vi "systemid-hardware-analyzer.vi"() -> ()   [LabVIEW 2012]
uses:
  <vilib>/addons/Control Design/_Utility/Model Viewer.llb/Model Viewer SubVI/cd_Draw Zero-Pole-Gain Equation (ZPK).vi
  <vilib>/imath/engines/lvmath2/RunTimeEngine/ErrorHandling/NIMS_Finalize Error.vi
  <vilib>/imath/engines/lvmath2/RunTimeEngine/Managers/WorkSpace/UID Generator.vi
  <vilib>/imath/engines/lvmath/Plug In/_Char/NIMS_CH_U8 2D to Character 2D.vi
  <vilib>/imath/engines/lvmath/Plug In/_Char/NIMS_CH_Character 2D to String 1D.vi
  <vilib>/imath/engines/lvmath2/RunTimeEngine/NodeEndStatement/NIMS_NodeEndStatement_Get Scalar.vi
  <instcachedir>/0/NIMS_NodeEndStatement_Get Scalar_DDDE03B66C1B40AEB228387CE0451FA8.lvgen/NIMS_NodeEndStatement_Get Scalar_DDDE03B66C1B40AEB228387CE0451FA8_000.vi
  <vilib>/imath/engines/lvmath2/RunTimeEngine/NodeEndStatement/NIMS_NodeEndStatement_Get Vector.vi
  <instcachedir>/0/NIMS_NodeEndStatement_Get Vector_2BE3967F82A04EDB90B65AFAEF9E88C9.lvgen/NIMS_NodeEndStatement_Get Vector_2BE3967F82A04EDB90B65AFAEF9E88C9_001.vi
  <instcachedir>/0/NIMS_NodeEndStatement_Get Vector_2BE3967F82A04EDB90B65AFAEF9E88C9.lvgen/NIMS_NodeEndStatement_Get Vector_2BE3967F82A04EDB90B65AFAEF9E88C9_003.vi
  <instcachedir>/0/NIMS_NodeEndStatement_Get Vector_2BE3967F82A04EDB90B65AFAEF9E88C9.lvgen/NIMS_NodeEndStatement_Get Vector_2BE3967F82A04EDB90B65AFAEF9E88C9_002.vi
  <vilib>/imath/engines/lvmath/Functions/Error Handling/MergeErrorsWrapper.vi
  <vilib>/imath/engines/lvmath2/RunTimeEngine/Managers/SymbolTable/Clear UID.vi
  <vilib>/imath/engines/lvmath2/RunTimeEngine/NodeEndStatement/NIMS_NodeEndStatement_Output.vi
  <instcachedir>/0/NIMS_NodeEndStatement_Output_53EC0D466D134D7ABD903AC30B43404B.lvgen/NIMS_NodeEndStatement_Output_53EC0D466D134D7ABD903AC30B43404B_001.vi
  <instcachedir>/0/NIMS_NodeEndStatement_Output_53EC0D466D134D7ABD903AC30B43404B.lvgen/NIMS_NodeEndStatement_Output_53EC0D466D134D7ABD903AC30B43404B_014.vi
  <instcachedir>/0/NIMS_NodeEndStatement_Output_53EC0D466D134D7ABD903AC30B43404B.lvgen/NIMS_NodeEndStatement_Output_53EC0D466D134D7ABD903AC30B43404B_005.vi
  <instcachedir>/0/NIMS_NodeEndStatement_Output_53EC0D466D134D7ABD903AC30B43404B.lvgen/NIMS_NodeEndStatement_Output_53EC0D466D134D7ABD903AC30B43404B_008.vi
  <vilib>/imath/engines/lvmath/Plug In/Control Design/BuiltInFunctions/ss/NIMS_CD_ss(A,B,C,D).vi
  <vilib>/imath/engines/lvmath2/RunTimeEngine/ArithmeticOperatorToken/NIMS_ArithmeticOperator_rightdiv.vi
  <instcachedir>/0/NIMS_ArithmeticOperator_rightdiv_C818BB5D803545678F946194135768CB.lvgen/NIMS_ArithmeticOperator_rightdiv_C818BB5D803545678F946194135768CB_000.vi
  <vilib>/imathl/engines/lvmath/Functions/Error Handling/Create Error.vi
  <vilib>/imath/engines/lvmath2/RunTimeEngine/ArithmeticOperatorToken/NIMS_ArithmeticOperator_minus.vi
  <instcachedir>/0/NIMS_ArithmeticOperator_minus_E353D3D62E0E432C853B0E64BA14CDF8.lvgen/NIMS_ArithmeticOperator_minus_E353D3D62E0E432C853B0E64BA14CDF8_003.vi
  <vilib>/imath/engines/lvmath/Plug In/Control Design/BuiltInFunctions/nyquist/NIMS_CD_[W,Mag,Pha]=nyquist(SS,[Winfo]).vi
  <vilib>/imath/engines/lvmath2/RunTimeEngine/RunTimeType/NIMS_RunTimeType_From StrictType (excl LVString).vi
  <instcachedir>/0/NIMS_RunTimeType_From StrictType (excl LVString)_AC52D965D0864706932D20A05968E122.lvgen/NIMS_RunTimeType_From StrictType (excl LVString)_AC52D965D0864706932D20A05968E122_000.vi
  <vilib>/imath/engines/lvmath2/RunTimeEngine/LocalVariableDefStatement/MC_LocalVariableDefStatement_Display.vi
  <instcachedir>/0/NIMS_ArithmeticOperator_rightdiv_C818BB5D803545678F946194135768CB.lvgen/NIMS_ArithmeticOperator_rightdiv_C818BB5D803545678F946194135768CB_004.vi
  <instcachedir>/0/NIMS_ArithmeticOperator_minus_E353D3D62E0E432C853B0E64BA14CDF8.lvgen/NIMS_ArithmeticOperator_minus_E353D3D62E0E432C853B0E64BA14CDF8_002.vi
  <vilib>/imath/engines/lvmath2/RunTimeEngine/BuiltInFunctions/min/1 input/NIMS_min(RM).vi
  <instcachedir>/0/NIMS_min(RM)_39359137F44A4A238B60DF61AC4DCB20.lvgen/NIMS_min(RM)_39359137F44A4A238B60DF61AC4DCB20_000.vi
  <vilib>/imath/engines/lvmath2/RunTimeEngine/BuiltInFunctions/mean/NIMS_RRow=mean(RM,I32).vi
  <vilib>/imath/engines/lvmath2/RunTimeEngine/BuiltInFunctions/max/1 input/NIMS_max(RM).vi
  <instcachedir>/0/NIMS_max(RM)_CB606D9E2D4C402AB2F89B43E5573F0F.lvgen/NIMS_max(RM)_CB606D9E2D4C402AB2F89B43E5573F0F_000.vi
  <vilib>/imath/engines/lvmath2/RunTimeEngine/BuiltInFunctions/findnz/NIMS_[1o]_findnz(GRowV).vi
  <instcachedir>/0/NIMS_[1o]_findnz(GRowV)_FE7C6D253574468A8FF8F3777E2F932A.lvgen/NIMS_[1o]_findnz(GRowV)_FE7C6D253574468A8FF8F3777E2F932A_000.vi
  <vilib>/imath/engines/lvmath2/RunTimeEngine/VariableToken/Read/NIMS_Get Elements - RV(_) - Check.vi
  <instcachedir>/0/NIMS_Get Elements - RV(_) - Check_09E565EE58C54071A799578B82C9999A.lvgen/NIMS_Get Elements - RV(_) - Check_09E565EE58C54071A799578B82C9999A_005.vi
  <vilib>/imath/engines/lvmath2/RunTimeEngine/VariableToken/Read/NIMS_Get Elements - SorM(_) - Check.vi
  <instcachedir>/0/NIMS_Get Elements - SorM(_) - Check_8FDA2664A675493882C25203DD903B51.lvgen/NIMS_Get Elements - SorM(_) - Check_8FDA2664A675493882C25203DD903B51_007.vi
  <vilib>/imath/engines/lvmath2/RunTimeEngine/BuiltInFunctions/max/1 input/NIMS_max(RV).vi
  <instcachedir>/0/NIMS_max(RV)_237633DB1D604D5BA7001287DF3C7957.lvgen/NIMS_max(RV)_237633DB1D604D5BA7001287DF3C7957_000.vi
  <vilib>/imath/engines/lvmath2/RunTimeEngine/BuiltInFunctions/min/1 input/NIMS_min(RV).vi
  <instcachedir>/0/NIMS_min(RV)_EE2DD3E2888846108C5160A664B67832.lvgen/NIMS_min(RV)_EE2DD3E2888846108C5160A664B67832_000.vi
  <vilib>/imath/engines/lvmath/Plug In/Control Design/BuiltInFunctions/zpk/NIMS_CD_zpk(zeros,poles,k,Ts).vi
  <vilib>/imath/engines/lvmath/Plug In/Control Design/BuiltInFunctions/nyquist/NIMS_CD_[W,Mag,Pha]=nyquist(ZPK,[Winfo]).vi
  <vilib>/imath/engines/lvmath2/RunTimeEngine/BuiltInFunctions/size/NIMS_I32Row=size(GRow).vi
  <instcachedir>/0/NIMS_I32Row=size(GRow)_E5C05C6B13124B29B774CC4F993D3C59.lvgen/NIMS_I32Row=size(GRow)_E5C05C6B13124B29B774CC4F993D3C59_000.vi
  <vilib>/imath/engines/lvmath2/RunTimeEngine/BuiltInFunctions/ones/NIMS_M=ones(I32V).vi
  <vilib>/imath/engines/lvmath2/RunTimeEngine/ReplaceToken/NIMS_Replace - Check Linear.vi
  <instcachedir>/0/NIMS_Replace - Check Linear_44ABB4D6A819426DBDF25CCE6827BF1D.lvgen/NIMS_Replace - Check Linear_44ABB4D6A819426DBDF25CCE6827BF1D_010.vi
  <vilib>/imath/engines/lvmath2/RunTimeEngine/ReplaceToken/NIMS_Replace - Size Check _(_)=S.vi
  <instcachedir>/0/NIMS_Replace - Size Check _(_)=S_5AC8AA27B9694BB9828B57BCF666F597.lvgen/NIMS_Replace - Size Check _(_)=S_5AC8AA27B9694BB9828B57BCF666F597_006.vi
  <vilib>/imath/engines/lvmath2/RunTimeEngine/ReplaceToken/NIMS_Replace - M(V)=S.vi
  <instcachedir>/0/NIMS_Replace - M(V)=S_5C546F19A34041D4875B70B08B385799.lvgen/NIMS_Replace - M(V)=S_5C546F19A34041D4875B70B08B385799_004.vi
  <instcachedir>/0/NIMS_I32Row=size(GRow)_E5C05C6B13124B29B774CC4F993D3C59.lvgen/NIMS_I32Row=size(GRow)_E5C05C6B13124B29B774CC4F993D3C59_001.vi
  <vilib>/imath/engines/lvmath2/RunTimeSupport/NIMS_Get Scalar_w Error.vi
  <instcachedir>/0/NIMS_Get Scalar_w Error_C4FC1D98B71F42F68E44AE98B50D76D1.lvgen/NIMS_Get Scalar_w Error_C4FC1D98B71F42F68E44AE98B50D76D1_010.vi
  <vilib>/imath/engines/lvmath2/RunTimeEngine/BuiltInFunctions/ones/NIMS_M=ones(I32,I32).vi
  <vilib>/imath/engines/lvmath2/RunTimeEngine/ErrorHandling/NIMS_Create Error From Enums.vi
  <vilib>/imath/engines/lvmath2/RunTimeEngine/BuiltInFunctions/num_to_str/NIMS_num_to_str(GM,I32).vi
  <instcachedir>/0/NIMS_num_to_str(GM,I32)_773DA44A11E3477FB6A93915E69D7E9F.lvgen/NIMS_num_to_str(GM,I32)_773DA44A11E3477FB6A93915E69D7E9F_000.vi
  <vilib>/imath/engines/lvmath/Plug In/_Char/NIMS_CH_String CV to Character 2D.vi
  <instcachedir>/0/NIMS_CH_String CV to Character 2D_B2E5264245B74746A343EBB64433A4F6.lvgen/NIMS_CH_String CV to Character 2D_B2E5264245B74746A343EBB64433A4F6_000.vi
  <vilib>/Utility/file.llb/Read From Spreadsheet File (DBL).vi
  <vilib>/measure/matone.llb/Extract Single Tone Information 1 Chan.vi
  <instcachedir>/0/NIMS_NodeEndStatement_Output_53EC0D466D134D7ABD903AC30B43404B.lvgen/NIMS_NodeEndStatement_Output_53EC0D466D134D7ABD903AC30B43404B_015.vi
  <vilib>/imath/engines/lvmath2/RunTimeEngine/BuiltInFunctions/sort/NIMS_[2o]_sort(RRowV,I32,Str).vi
  <instcachedir>/0/NIMS_[2o]_sort(RRowV,I32,Str)_EF5336185A744094BB84441B99878C05.lvgen/NIMS_[2o]_sort(RRowV,I32,Str)_EF5336185A744094BB84441B99878C05_000.vi
  <vilib>/imath/engines/lvmath2/RunTimeEngine/BuiltInFunctions/length/NIMS_length(GV).vi
  <instcachedir>/0/NIMS_length(GV)_08A3D13377FD4E4B96F5795FBF3698FA.lvgen/NIMS_length(GV)_08A3D13377FD4E4B96F5795FBF3698FA_002.vi
  <vilib>/measure/NI_MAPro.lvlib
  <vilib>/addons/Control Design/_Utility/NI_CD_Model Viewer.lvlib
  <vilib>/imath/engines/lvmath2/RunTimeEngine/Managers/SymbolTable/NIMS_WorkSpace.lvlib
panel:
  out "Maximum Khw":dbl
  out "Minimum Khw":dbl
  out "Average Khw (Nm/V)":dbl
  in  "z":dbl=-1.0 step=0.01
  in  "p":dbl=-0.1 step=0.01
  in  "k":dbl=-0.35 step=0.01
  in  "Tab Control":T1(tab)
  out "InputSets":cluster{dbl[], dbl[]}(graph)
  out "Voltage->Angle Phase":cluster{dbl[], dbl[]}(graph) caption="Gain"
  out "Voltage->Angle Gain":cluster{dbl[], dbl[]}(graph) caption="Gain"
  out "Voltage->Torque Phase":cluster{dbl[], dbl[]}[](graph) caption="Gain"
  out "Voltage->Torque Gain":cluster{dbl[], dbl[]}[](graph) caption="Gain"
  out "Torque->Angle Phase":cluster{dbl[], dbl[]}(graph) caption="Gain"
  out "Torque->Angle Gain":cluster{dbl[], dbl[]}(graph) caption="Gain"
  out "Processed Input Measurement":waveform(dbl)(graph)
  out "Raw Input Measurement":waveform(dbl)(graph)
  out "Processed Output Measurement":waveform(dbl)(graph)
  out "Raw Output Measurement":waveform(dbl)(graph)
  in  "Damping Coefficient (Nm-s/rad)":dbl=0.018
  in  "Rotational Inertia (kg-m^2)":dbl=0.019225
  in  "Data Listbox":i32(listbox)
  out "Data":T2(array[cluster])
  # "Use to fit a Lead-Lag controller to the Voltage->Torque data:"
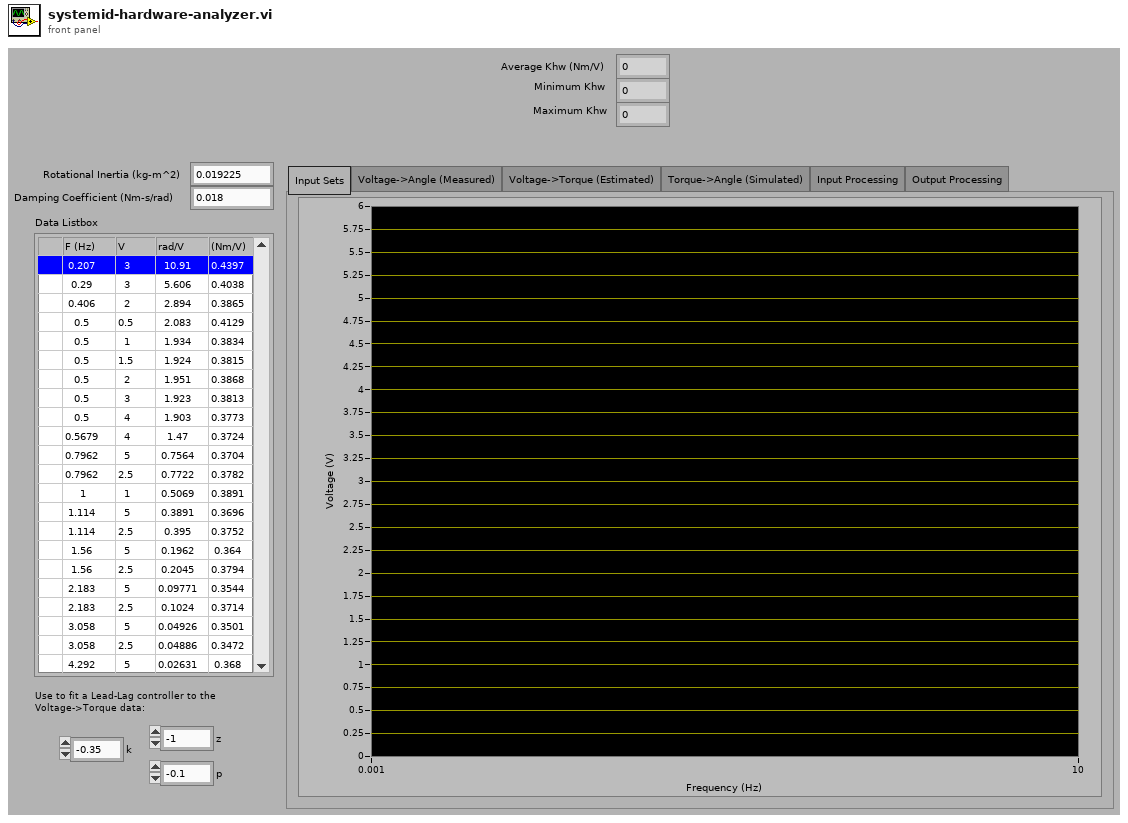
[diagram p1: front panel]
types:
  T1 = enum32{"Input Sets", "Voltage->Angle (Measured)", "Voltage->Torque (Estimated)", "Torque->Angle (Simulated)", "Input Processing", "Output Processing"}
  T2 = cluster{"Enabled":bool, "U Amp. (V)":dbl, "A Gain(rad/V)":dbl, "T Gain (Nm/V)":dbl, "Frequency (Hz)":dbl, "A Phase(rad)":dbl, "T Phase (rad)":dbl, "Sample Period (s)":dbl, "Input Data (V)":waveform(dbl), "Output Data (rad)":waveform(dbl), "U Phase (deg)":dbl, "Y Amp. (rad)":dbl, "Y Phase (rad)":dbl, "Input Fit (V)":waveform(dbl), "Output Fit(rad)":waveform(dbl)}[]
  T3 = enum32{"none", "input signal", "detected signal", "residual signal"}
  T4 = cluster{"Enabled":bool, "U Amp. (V)":dbl, "A Gain(rad/V)":dbl, "T Gain (Nm/V)":dbl, "Frequency (Hz)":dbl, "A Phase(rad)":dbl, "T Phase (rad)":dbl, "Sample Period (s)":dbl, "Input Data (V)":waveform(dbl), "Output Data (rad)":waveform(dbl), "U Phase (deg)":dbl, "Y Amp. (rad)":dbl, "Y Phase (rad)":dbl, "Input Fit (V)":waveform(dbl), "Output Fit(rad)":waveform(dbl)}
  T5 = cluster{"first row[0]":dbl, "first row[1]":dbl, "first row[2]":dbl}
  T6 = cluster{"exported time signal":waveform(dbl), "exported spectrum (dB)":cluster{"f0":dbl, "df":dbl, "dB Spectrum (Hann)":dbl[]}}
  T7 = typedef "NI_LinSys_Model Typedefs.lvlib/CD Zero-Pole-Gain Model (MIMO).ctl" = cluster{"properties":T8, "zero-pole-gain(s)":T9[][]}
  T8 = typedef "NI_LinSys_Model Typedefs.lvlib/CD General Elements.ctl" = cluster{"Model name":string, "Input names":string[], "Output names":string[], "Input Delays":dbl[], "Output Delays":dbl[], "Sampling Time":dbl, "Notes":string}
  T9 = typedef "NI_LinSys_Model Typedefs.lvlib/CD Zero-Pole-Gain Model (SISO).ctl" = cluster{"Gain":dbl, "Zeros":cdb[], "Poles":cdb[], "delay":dbl}
  T10 = cluster{"FpiEnabled":dbl[], "aGainEnabled":dbl[]}
  T11 = cluster{"FpiEnabled":dbl[], "aPhaseEnabled":dbl[]}
  T12 = cluster{"FpiEnabled":dbl[], "tGainEnabled":dbl[]}
  T13 = cluster{"FpiEnabled":dbl[], "tPhaseEnabled":dbl[]}
  T14 = cluster{"sysFreq":dbl[], "motPhaseClipped":dbl[]}
  T15 = cluster{"sysFreq":dbl[], "sysPhaseClipped":dbl[]}
  T16 = cluster{"sysFreq":dbl[], "motGainClipped":dbl[]}[]
  T17 = cluster{"sysFreq":dbl[], "motPhaseClipped":dbl[]}[]
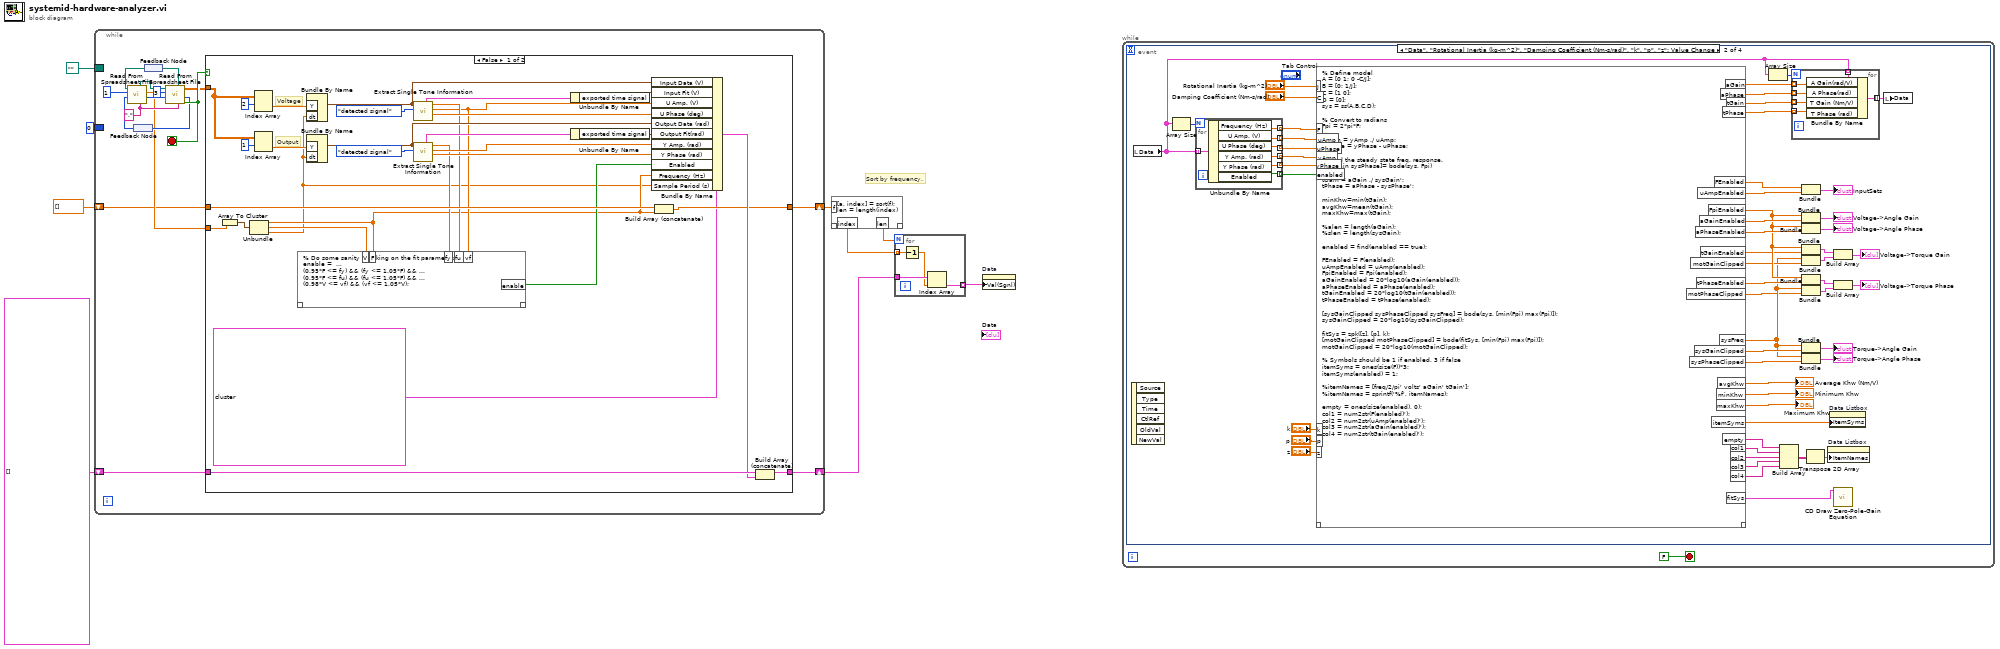
[diagram p0: block diagram]
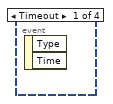
[diagram p2: hidden frame]
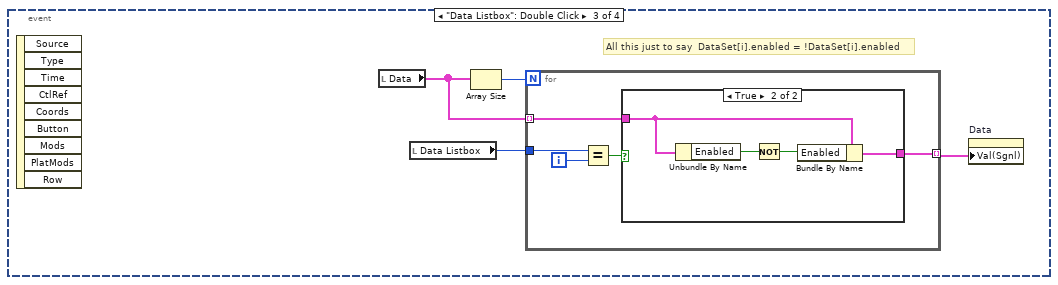
[diagram p3: hidden frame]
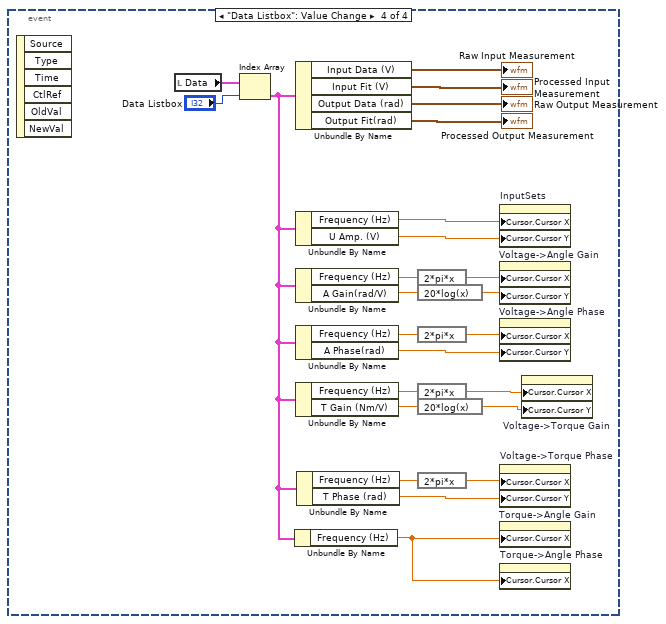
[diagram p5: hidden frame]
diagram:
  # "Sort by frequency."
  n1 = while {
    shift-right: [w24] -> w6
    shift-left: T2 [] -> [w25]
    shift-right: [w11] -> w9
    shift-left: dbl[] [] -> [w12]
    border: 0 ("mark after read (chars.)") -> [_]
    border: path "" ("new file path (Not A Path if cancelled)") -> [_]
    stop <- w21 stop-if-true
    w20 = "," ("delimiter (\\t)")
    n2 = feedback #1() -> (w22:i32)
    n3 = feedback #2() -> (w15:path)
    n4 = call-poly <vilib>:"Read From Spreadsheet File.vi"("delimiter (\\t)"=w20, "start of read offset (chars.:0)"=w22, "number of rows (all:-1)"=1, "file path (dialog if empty)"=w15) -> ("mark after read (chars.)"=w19:i32, "first row"=w13:dbl[], "new file path (Not A Path if cancelled)"=w17:path)  [unwired: 3 in, 2 out]
    n5 = call-poly <vilib>:"Read From Spreadsheet File.vi"("delimiter (\\t)"=w20, "start of read offset (chars.:0)"=w19, "number of rows (all:-1)"=3, "file path (dialog if empty)"=w17) -> ("EOF?"=w21:bool, "mark after read (chars.)"=w18:i32, "all rows"=w14:dbl[][], "new file path (Not A Path if cancelled)"=w16:path)  [unwired: 3 in, 1 out]
    n6 = feedback-in #1(w18) -> ()
    n7 = feedback-in #2(w16) -> ()
    n8 = case shown="False" w21 {
      tunnel: w25 -> [w56 w138]
      tunnel: [w55 w138] -> w24
      tunnel: w14 -> [w53 _]
      tunnel: w13 -> [w50 _]
      tunnel: w12 -> [w48 w137]
      tunnel: [w47 w137] -> w11
      frame False {
        # "Voltage"
        # "Output"
        n9 = Array To Cluster(array=w50) -> (cluster=w49:T5)
        n10 = Unbundle(w49) -> ("first row[0]"=w27:dbl, "first row[1]"=w30:dbl, "first row[2]"=w26:dbl)
        n11 = Index Array(array=w53, index (row)=2) -> (element=w45:dbl[])  [unwired: 1 in]
        n12 = Index Array(array=w53, index (row)=1) -> (element=w46:dbl[])  [unwired: 1 in]
        n13 = Bundle By Name("Y"=w45, "dt"=w26) -> (w37:waveform(dbl))  [unwired: 1 in]
        n14 = Bundle By Name("Y"=w46, "dt"=w26) -> (w38:waveform(dbl))  [unwired: 1 in]
        n15 = call-poly <vilib>:"Extract Single Tone Information.vi"("export mode"=T3."detected signal" ("export signals"), "time signal in"=w37) -> ("detected phase (deg)"=w39:dbl, "detected amplitude"=w29:dbl, "detected frequency"=w32:dbl, "exported signals"=w42:T6)  [unwired: 4 in, 2 out]
        n16 = call-poly <vilib>:"Extract Single Tone Information.vi"("export mode"=T3."detected signal" ("export signals"), "time signal in"=w38) -> ("detected phase (deg)"=w33:dbl, "detected amplitude"=w34:dbl, "detected frequency"=w31:dbl, "exported signals"=w35:T6)  [unwired: 4 in, 2 out]
        n17 = mathscript code="% Do some sanity checking on the fit parameters\nenable =  ...\n(0.95*F <= fy) && (fy <= 1.05*F) && ...\n(0.95*F <= fu) && (fu <= 1.05*F) && ...\n(0.98*V <= vf) && (vf <= 1.05*V);"("F"=w27, "fu"=w32, "fy"=w31, "V"=w30, "vf"=w29) -> ("enable"=w28:bool)  [unwired: 1 in, 1 out]
        n18 = Unbundle By Name(w42) -> ("exported time signal"=w41:waveform(dbl))
        n19 = Unbundle By Name(w35) -> ("exported time signal"=w36:waveform(dbl))
        n20 = Bundle By Name(cluster=T4 {"Enabled"=TRUE, "U Amp. (V)"=0.0, "A Gain(rad/V)"=0.0, "T Gain (Nm/V)"=0.0, "Frequency (Hz)"=0.0, "A Phase(rad)"=0.0, "T Phase (rad)"=0.0, "Sample Period (s)"=0.0, "Input Data (V)"={"t0"=timestamp(0 s since 1904-01-01), "dt"=1.0, "Y"=[]}, "Output Data (rad)"={"t0"=timestamp(0 s since 1904-01-01), "dt"=1.0, "Y"=[]}, "U Phase (deg)"=0.0, "Y Amp. (rad)"=0.0, "Y Phase (rad)"=0.0, "Input Fit (V)"={"t0"=timestamp(0 s since 1904-01-01), "dt"=1.0, "Y"=[]}, "Output Fit(rad)"={"t0"=timestamp(0 s since 1904-01-01), "dt"=1.0, "Y"=[]}}, "Input Data (V)"=w37, "Input Fit (V)"=w41, "U Amp. (V)"=w29, "U Phase (deg)"=w39, "Output Data (rad)"=w38, "Output Fit(rad)"=w36, "Y Amp. (rad)"=w34, "Y Phase (rad)"=w33, "Enabled"=w28, "Frequency (Hz)"=w27, "Sample Period (s)"=w26) -> (w54:T4)
        n21 = Build Array (concatenate)(w48, w27) -> (w47:dbl[])
        n22 = Build Array (concatenate)(w56, w54) -> (w55:T2)
      }
      frame True {
      }
    }
  }
  n23 = mathscript code="[a, index] = sort(f);\nlen = length(index)"("f"=w9) -> ("index"=w7:dbl[], "len"=w8:dbl)  [unwired: 1 in, 1 out]
  n24 = for {
    N: w8 -> [_]
    tunnel: w7 -> [w139] mode=indexing
    tunnel: w6 -> [w142]
    tunnel: [w141] -> w2 mode=indexing
    n25 = Decrement(x=w139) -> (x-1=w140:dbl)
    n26 = Index Array(array=w142, index=w140) -> (element=w141:T4)
  }
  n27 = property on="Data" class="Arr (strict)"("Val(Sgnl)"=w2) -> ()  [unwired: 2 in, 2 out]
  n28 = while {
    stop <- FALSE stop-if-true
    n29 = event shown="[1] \"Data\", \"Rotational Inertia (kg-m^2)\", \"Damping Coefficient (Nm-s/rad)\", \"k\", \"p\", \"z\": Value Change" {
      selector: _ -> [_ _ _ _]
      dyn-events: _ -> [_ _ _ _]
      timeout: _ -> [_ _ _ _]
      event Timeout {
        n30 = event-data() -> ()  [unwired: 1 in, 2 out]
      }
      event "Data", "Rotational Inertia (kg-m^2)", "Damping Coefficient (Nm-s/rad)", "k", "p", "z": Value Change {
        n31 = event-data() -> ()  [unwired: 1 in, 6 out]
        n32 = local read "Data"() -> (w187:T2)
        n33 = Array Size(array=w187) -> (size(s)=w197:i32)
        n34 = for {
          N: w197 -> [_]
          tunnel: w187 -> [w781] mode=indexing
          tunnel: [w780] -> w191 mode=indexing
          tunnel: [w779] -> w196 mode=indexing
          tunnel: [w778] -> w195 mode=indexing
          tunnel: [w777] -> w194 mode=indexing
          tunnel: [w776] -> w193 mode=indexing
          tunnel: [w775] -> w192 mode=indexing
          n35 = Unbundle By Name(w781) -> ("Frequency (Hz)"=w775:dbl, "U Amp. (V)"=w776:dbl, "U Phase (deg)"=w777:dbl, "Y Amp. (rad)"=w778:dbl, "Y Phase (rad)"=w779:dbl, "Enabled"=w780:bool)
        }
        n36 = mathscript code="% Define model\nA = [0 1; 0 -C/J];\nB = [0; 1/J]; \nC = [1 0];\nD = [0];\nsys = ss(A,B,C,D);\n\n% Convert to radians\nFpi = 2*pi*F;   \n\naGain = yAmp ./ uAmp;\naPhase = yPhase - uPhase;\n\n% Find the steady state freq. response.\n[sysGain sysPhase]= bode(sys, Fpi)\n\ntGain = aGain ./ sysGain';\ntPhase = aPhase - sysPhase';\n\nminKhw=min(tGain);\navgKhw=mean(tGain);\nmaxKhw=max(tGain);\n\n%alen = length(aGain);\n%slen = length(sysGain);\n\nenabled = find(enabled == true);\n\nFEnabled = F(enabled);\nuAmpEnabled = uAmp(enabled);\nFpiEnabled = Fpi(enabled);\naGainEnabled = 20*log10(aGain(enabled));\naPhaseEnabled = aPhase(enabled);\ntGainEnabled = 20*log10(tGain(enabled));\ntPhaseEnabled = tPhase(enabled);\n\n[sysGainClipped sysPhaseClipped sysFreq] = bode(sys, [min(Fpi) max(Fpi)]);\nsysGainClipped = 20*log10(sysGainClipped);\n\nfitSys = zpk([z], [p], k);\n[motGainClipped motPhaseClipped] = bode(fitSys, [min(Fpi) max(Fpi)]);\nmotGainClipped = 20*log10(motGainClipped);\n\n% Symbols should be 1 if enabled, 3 if false\nitemSyms = ones(size(F))*3;\nitemSyms(enabled) = 1;\n\n%itemNames = [freq/2/pi' volts' aGain' tGain'];\n%itemNames = sprintf('%f', itemNames);\n\nempty = ones(size(enabled), 0);\ncol1 = num2str(F(enabled)');\ncol2 = num2str(uAmp(enabled)');\ncol3 = num2str(aGain(enabled)');\ncol4 = num2str(tGain(enabled)');"("F"=w192, "uAmp"=w193, "uPhase"=w194, "yAmp"=w195, "yPhase"=w196, "enabled"=w191, "J"="Rotational Inertia (kg-m^2)", "C"="Damping Coefficient (Nm-s/rad)", "k"="k", "p"="p", "z"="z") -> ("aGain"=w186:dbl[], "aPhase"=w185:dbl[], "tGain"=w184:dbl[], "tPhase"=w183:dbl[], "col1"=w179:string[], "col2"=w180:string[], "col3"=w177:string[], "col4"=w176:string[], "itemSyms"=w181:dbl[], "empty"=w178:string[], "FpiEnabled"=w165:dbl[], "aGainEnabled"=w172:dbl[], "aPhaseEnabled"=w171:dbl[], "FEnabled"=w168:dbl[], "uAmpEnabled"=w169:dbl[], "tGainEnabled"=w163:dbl[], "tPhaseEnabled"=w164:dbl[], "sysFreq"=w152:dbl[], "sysGainClipped"=w162:dbl[], "sysPhaseClipped"=w161:dbl[], "motGainClipped"=w156:dbl[], "motPhaseClipped"=w151:dbl[], "fitSys"=w147:T7, "avgKhw"=→"Average Khw (Nm/V)":dbl, "minKhw"=→"Minimum Khw":dbl, "maxKhw"=→"Maximum Khw":dbl)  [unwired: 1 in, 1 out]
        n37 = Array Size(array=w187) -> (size(s)=w188:i32)
        n38 = Build Array(w178, w179, w180, w177, w176) -> (w174:string[][])
        n39 = for {
          N: w188 -> [_]
          tunnel: w187 -> [w203] mode=indexing
          tunnel: w186 -> [w202] mode=indexing
          tunnel: w185 -> [w201] mode=indexing
          tunnel: w184 -> [w200] mode=indexing
          tunnel: w183 -> [w199] mode=indexing
          tunnel: [w198] -> w182 mode=indexing
          n40 = Bundle By Name(cluster=w203, "A Gain(rad/V)"=w202, "A Phase(rad)"=w201, "T Gain (Nm/V)"=w200, "T Phase (rad)"=w199) -> (w198:T4)
        }
        n41 = Bundle("FEnabled"=w168, "uAmpEnabled"=w169) -> (→"InputSets":cluster{"FEnabled":dbl[], "uAmpEnabled":dbl[]})  [unwired: 1 in]
        n42 = Bundle("FpiEnabled"=w165, "aGainEnabled"=w172) -> (→"Voltage->Angle Gain":T10)  [unwired: 1 in]
        n43 = Bundle("FpiEnabled"=w165, "aPhaseEnabled"=w171) -> (→"Voltage->Angle Phase":T11)  [unwired: 1 in]
        n44 = Bundle("FpiEnabled"=w165, "tGainEnabled"=w163) -> (w155:T12)  [unwired: 1 in]
        n45 = Bundle("sysFreq"=w152, "motGainClipped"=w156) -> (w154:cluster{"sysFreq":dbl[], "motGainClipped":dbl[]})  [unwired: 1 in]
        n46 = Bundle("FpiEnabled"=w165, "tPhaseEnabled"=w164) -> (w149:T13)  [unwired: 1 in]
        n47 = Bundle("sysFreq"=w152, "motPhaseClipped"=w151) -> (w150:T14)  [unwired: 1 in]
        n48 = Bundle("sysFreq"=w152, "sysGainClipped"=w162) -> (→"Torque->Angle Gain":cluster{"sysFreq":dbl[], "sysGainClipped":dbl[]})  [unwired: 1 in]
        n49 = Bundle("sysFreq"=w152, "sysPhaseClipped"=w161) -> (→"Torque->Angle Phase":T15)  [unwired: 1 in]
        n50 = Transpose 2D Array(2D array=w174) -> (transposed array=w175:string[][])
        n51 = property on="Data Listbox" class="MCListbox (strict)"("ItemNames"=w175) -> ()  [unwired: 2 in, 2 out]
        n52 = property on="Data Listbox" class="MCListbox (strict)"("ItemSyms"=w181) -> ()  [unwired: 2 in, 2 out]
        n53 = Build Array(w155, w154) -> (→"Voltage->Torque Gain":T16)
        n54 = Build Array(w149, w150) -> (→"Voltage->Torque Phase":T17)
        n55 = call-poly <vilib>:"CD Draw Zero-Pole-Gain Equation.vi"("Zero-Pole-Gain Model"=w147) -> ()  [unwired: 8 in, 3 out]
        n56 = local write "Data"(w182) -> ()
      }
      event "Data Listbox": Double Click {
        # "All this just to say  DataSet[i].enabled = !DataSet[i].enabled"
        n57 = event-data() -> ()  [unwired: 1 in, 9 out]
        n58 = local read "Data"() -> (w784:T2)
        n59 = local read "Data Listbox"() -> (w783:i32)
        n60 = Array Size(array=w784) -> (size(s)=w785:i32)
        n61 = for {
          N: w785 -> [_]
          tunnel: w784 -> [w787] mode=indexing
          tunnel: w783 -> [w788]
          tunnel: [w786] -> w782 mode=indexing
          i -> [w789]
          n62 = Equal?(x=w788, y=w789) -> (x = y?=w790:bool)
          n63 = case shown="True" w790 {
            tunnel: w787 -> [w791 w795]
            tunnel: [w791 w792] -> w786
            frame False {
            }
            frame True {
              n64 = Unbundle By Name(w795) -> ("Enabled"=w794:bool)
              n65 = Not(x=w794) -> (.not. x?=w793:bool)
              n66 = Bundle By Name(cluster=w795, "Enabled"=w793) -> (w792:T4)
            }
          }
        }
        n67 = property on="Data" class="Arr (strict)"("Val(Sgnl)"=w782) -> ()  [unwired: 2 in, 2 out]
      }
      event "Data Listbox": Value Change {
        n68 = event-data() -> ()  [unwired: 1 in, 6 out]
        n69 = local read "Data"() -> (w819:T2)
        n70 = Index Array(array=w819, index="Data Listbox") -> (element=w810:T4)
        n71 = Unbundle By Name(w810) -> ("Frequency (Hz)"=w809:dbl)
        n72 = Unbundle By Name(w810) -> ("Input Data (V)"=→"Raw Input Measurement":waveform(dbl), "Input Fit (V)"=→"Processed Input Measurement":waveform(dbl), "Output Data (rad)"=→"Raw Output Measurement":waveform(dbl), "Output Fit(rad)"=→"Processed Output Measurement":waveform(dbl))
        n73 = Unbundle By Name(w810) -> ("Frequency (Hz)"=w813:dbl, "U Amp. (V)"=w812:dbl)
        n74 = Unbundle By Name(w810) -> ("Frequency (Hz)"=w804:dbl, "A Gain(rad/V)"=w808:dbl)
        n75 = Unbundle By Name(w810) -> ("Frequency (Hz)"=w797:dbl, "A Phase(rad)"=w811:dbl)
        n76 = Unbundle By Name(w810) -> ("Frequency (Hz)"=w798:dbl, "T Gain (Nm/V)"=w806:dbl)
        n77 = Unbundle By Name(w810) -> ("Frequency (Hz)"=w801:dbl, "T Phase (rad)"=w802:dbl)
        n78 = expression code="2*pi*x"(w804) -> (w803:dbl)
        n79 = expression code="20*log(x)"(w808) -> (w807:dbl)
        n80 = expression code="2*pi*x"(w797) -> (w796:dbl)
        n81 = expression code="2*pi*x"(w798) -> (w799:dbl)
        n82 = expression code="20*log(x)"(w806) -> (w805:dbl)
        n83 = expression code="2*pi*x"(w801) -> (w800:dbl)
        n84 = property on="InputSets" class="XYGraph (strict)"("Cursor.Cursor X"=w813, "Cursor.Cursor Y"=w812) -> ()  [unwired: 2 in, 2 out]
        n85 = property on="Voltage->Angle Gain" class="XYGraph (strict)"("Cursor.Cursor X"=w803, "Cursor.Cursor Y"=w807) -> ()  [unwired: 2 in, 2 out]
        n86 = property on="Voltage->Angle Phase" class="XYGraph (strict)"("Cursor.Cursor X"=w796, "Cursor.Cursor Y"=w811) -> ()  [unwired: 2 in, 2 out]
        n87 = property on="Voltage->Torque Phase" class="XYGraph (strict)"("Cursor.Cursor X"=w800, "Cursor.Cursor Y"=w802) -> ()  [unwired: 2 in, 2 out]
        n88 = property on="Torque->Angle Gain" class="XYGraph (strict)"("Cursor.Cursor X"=w809) -> ()  [unwired: 2 in, 2 out]
        n89 = property on="Torque->Angle Phase" class="XYGraph (strict)"("Cursor.Cursor X"=w809) -> ()  [unwired: 2 in, 2 out]
        n90 = property on="Voltage->Torque Gain" class="XYGraph (strict)"("Cursor.Cursor X"=w799, "Cursor.Cursor Y"=w805) -> ()  [unwired: 2 in, 2 out]
      }
    }
  }
